vi "Receive Signal DBL.vi"(8 "error in":errorcluster, 10 "Signal Name":string, 11 "DBC Communication in":refnum<class "DBC Communication.lvclass">) -> (0 "error out":errorcluster, 2 "Value":dbl, 3 "DBC Communication out":refnum<class "DBC Communication.lvclass">)   [LabVIEW 2024, in "DBC Communication.lvclass"]
uses:
  DBC Communication.lvclass
  DBC Communication.lvclass/DBC Communication.ctl
  <vilib>/xnet/xnet.llb/XNET Frame Type CAN.ctl
  Devices/PCAN/CAN Message/CAN Message.lvclass
  c9a96274-a027-4ccf-b481-50e0b552ac68.vi
  Interfaces/ICommunicate/ICommunicate.lvclass
  <vilib>/xnet/xnet.llb/XNET Convert (Frame CAN to Signal).vi
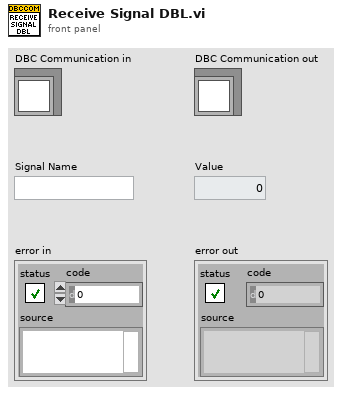
[diagram p1: front panel]
types:
  T1 = typedef "XNET Frame Type CAN.ctl" = u8
  T2 = cluster{"timestamp":timestamp, "payload":u8[], "identifier":u32, "type":T1, "extended?":bool, "echo?":bool}
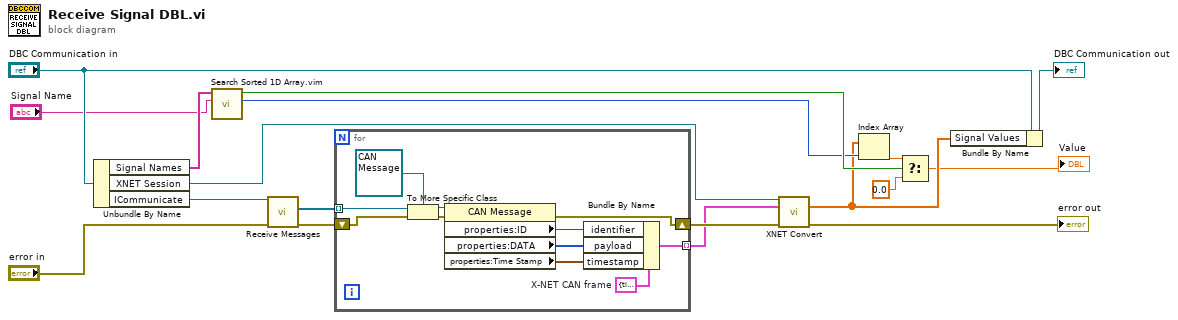
[diagram p0: block diagram]
diagram:
  n1 = Unbundle By Name("DBC Communication in") -> ("Signal Names"=w8:string[], "XNET Session"=w15:refnum<k21>, "ICommunicate"=w16:refnum<class "ICommunicate.lvclass">)
  n2 = call "Search Sorted 1D Array.vim"("element"="Signal Name", "sorted 1D array"=w8) -> ("nearest index"=w4:i32, "found?"=w6:bool)  [unwired: 8 in]
  n3 = call-dynamic "Receive Messages.vi"("error in"="error in", "ICommunicate in"=w16) -> ("error out"=w12:errorcluster, "Messages"=w14:refnum<class "IMessage.lvclass">[])  [unwired: 7 in, 1 out]
  n4 = for {
    tunnel: w14 -> [w28] mode=indexing
    shift-right: [w20] -> w11
    shift-left: w12 -> [w26]
    tunnel: [w19] -> w10 mode=indexing
    w29 = T2 {"timestamp"=timestamp(0 s since 1904-01-01), "payload"=[], "identifier"=0, "type"=0, "extended?"=FALSE, "echo?"=FALSE}  # X-NET CAN frame
    n5 = To More Specific Class(target class=refnum<class "CAN Message.lvclass"> refnum ("PCAN.lvlib:CAN Message"), reference=w28, error in=w26) -> (specific class reference=w24:refnum<class "CAN Message.lvclass">, error out=w25:errorcluster)
    n6 = property class="CAN Message"(reference=w24, error in=w25) -> (error out=w20:errorcluster, "properties:ID"=w23:u32, "properties:DATA"=w22:u8[], "properties:Time Stamp"=w21:timestamp)  [unwired: 1 out]
    n7 = Bundle By Name(cluster=w29, "identifier"=w23, "payload"=w22, "timestamp"=w21) -> (w19:T2)
  }
  n8 = call-poly <vilib>:"XNET Convert.vi"("session in"=w15, "frame data"=w10, "error in (no error)"=w11) -> ("signal data"=w2:dbl[], "error out"=→"error out":errorcluster)  [unwired: 10 in, 1 out]
  n9 = Index Array(array=w2, index=w4) -> (element=w5:dbl)
  n10 = Select(t=w5, s=w6, f=0.0) -> (s? t:f=→"Value":dbl)
  n11 = Bundle By Name(cluster="DBC Communication in", "Signal Values"=w2) -> (→"DBC Communication out":refnum<class "DBC Communication.lvclass">)
